vi "MainCamera_connect.vi"() -> ()   [LabVIEW 2018]
panel:
  out "error out":errorcluster
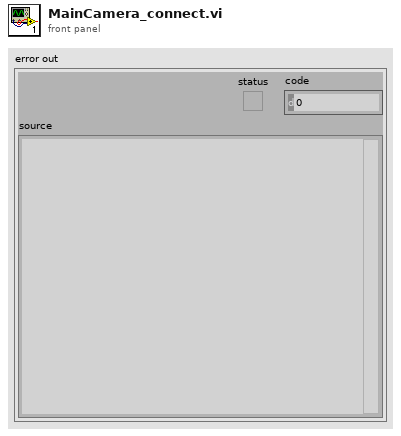
[diagram p1: front panel]
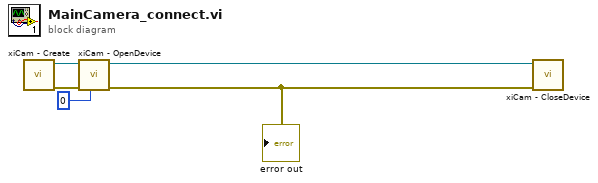
[diagram p0: block diagram]
diagram:
  n1 = call "xiCam - Create.vi"() -> ("error out"=w4:errorcluster, "new xiCam"=w5:refnum<k24>)  [unwired: 10 in]
  n2 = call "xiCam - OpenDevice.vi"("DevID"=0, "error in (no error)"=w4, "xiCam In"=w5) -> ("error out"=w1:errorcluster, "xiCam Out"=w2:refnum<k24>)  [unwired: 7 in]
  "error out" <- w1
  n3 = call "xiCam - CloseDevice.vi"("error in (no error)"=w1, "xiCam In"=w2) -> ()  [unwired: 9 in, 1 out]
